vi "Write Ramp Parameters.vi"(8 "error in (no error)":errorcluster, 10 "ramp parameters":T1 {"durations [s]"."ramp-down" format="%.2p"; "durations [s]"."transition" format="%.2p"; "durations [s]"."ramp-up" format="%.2p"}, 11 "signal configuration":refnum<class "SV Signal.lvclass">) -> (0 "error out":errorcluster, 3 "signal configuration":refnum<class "SV Signal.lvclass">)   [LabVIEW 2017, in "SV Signal.lvclass"]
uses:
  <vilib>/addons/_NISVFA/_Generation/Signal Generation/SV Signal/SV Signal.lvclass
  <vilib>/addons/_NISVFA/_Generation/Signal Generation/SV Signal/SV Signal.lvclass/SV Signal.ctl
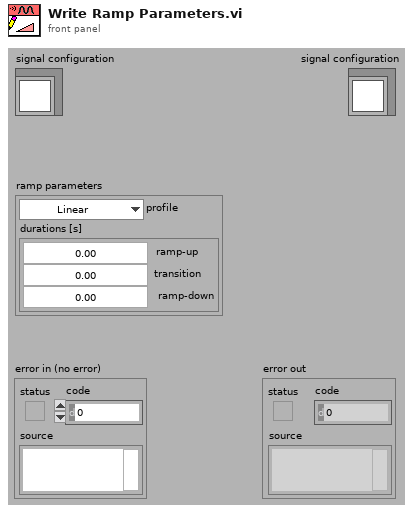
[diagram p1: front panel]
types:
  T1 = cluster{"profile":enum16{"Linear", "Half cosine"}, "durations [s]":cluster{"ramp-up":dbl, "transition":dbl, "ramp-down":dbl}}
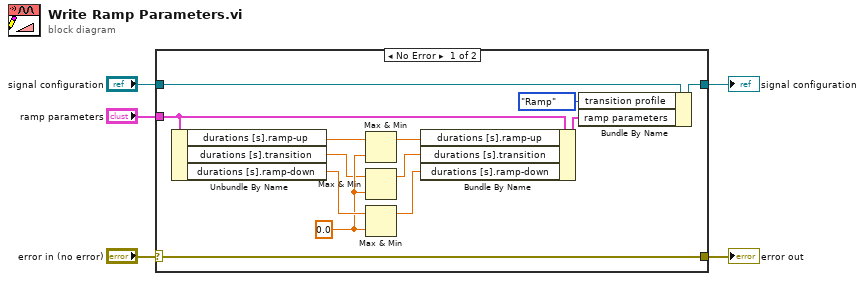
[diagram p0: block diagram]
diagram:
  n1 = case shown="No Error" "error in (no error)" {
    selector: "error in (no error)" -> [w18 w19]
    tunnel: [w18 w19] -> w4
    tunnel: [w16 w20] -> w2
    tunnel: "signal configuration" -> [w17 w20]
    tunnel: "ramp parameters" -> [w12 _]
    frame No Error {
      w8 = 0.0 ("y")
      n2 = Unbundle By Name(w12) -> ("durations [s].ramp-up"=w13:dbl, "durations [s].transition"=w6:dbl, "durations [s].ramp-down"=w14:dbl)
      n3 = Max & Min(x=w13, y=w8) -> (max(x,y)=w10:dbl)  [unwired: 1 out]
      n4 = Max & Min(x=w6, y=w8) -> (max(x,y)=w7:dbl)  [unwired: 1 out]
      n5 = Max & Min(x=w14, y=w8) -> (max(x,y)=w9:dbl)  [unwired: 1 out]
      n6 = Bundle By Name(cluster=w12, "durations [s].ramp-up"=w10, "durations [s].transition"=w7, "durations [s].ramp-down"=w9) -> (w11:T1)
      n7 = Bundle By Name(cluster=w17, "transition profile"=enum16{"Immediate", "Next optimum", "Ramp"}."Ramp", "ramp parameters"=w11) -> (w16:refnum<class "SV Signal.lvclass">)
    }
    frame Error {
    }
  }
  "error out" <- w4
  "signal configuration" <- w2
